vi "Find HTML Help Workshop Installation.vi"(8 "error in (no error)":errorcluster, 11 "Help Path":path) -> (0 "error out":errorcluster, 3 "Installation Path":string)   [LabVIEW 2015, in "HTML Help File Tools.lvlib"]
uses:
  HTML Help File Tools.lvlib
  <vilib>/registry/registry.llb/Registry RtKey.ctl
  <vilib>/registry/registry.llb/Registry SAM.ctl
  <vilib>/registry/registry.llb/Read Registry Value Simple STR.vi
  Log FGV Operation Modes.ctl
  Error Location.ctl
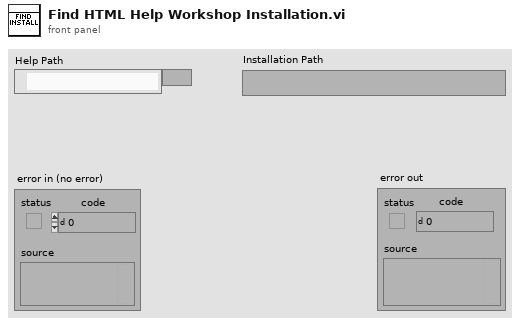
[diagram p1: front panel]
types:
  T1 = typedef "HTML Help File Tools.lvlib/Error Location.ctl" = enum16{"Delete tmp", "Compile HHP", "Find Install", "Create tmp", "Create HHP", "Find Help"}
  T2 = typedef "HTML Help File Tools.lvlib/Log FGV Operation Modes.ctl" = enum16{"Close", "Write", "Open File"}
  T3 = typedef "Registry SAM.ctl" = enum32{"KEY_QUERY_VALUE", "KEY_SET_VALUE", "KEY_CREATE_SUB_KEY", "KEY_ENUMERATE_SUB_KEYS", "KEY_NOTIFY", "KEY_CREATE_LINK", "KEY_READ", "KEY_WRITE", "KEY_ALL_ACCESS", "KEY_READ | KEY_WRITE"}
  T4 = typedef "Registry RtKey.ctl" = enum32{"HKEY_CLASSES_ROOT", "HKEY_CURRENT_USER", "HKEY_LOCAL_MACHINE", "HKEY_USERS", "HKEY_PERFORMANCE_DATA", "HKEY_CURRENT_CONFIG", "HKEY_DYN_DATA"}
  T5 = typedef "Registry refnum.ctl" = refnum<k1>
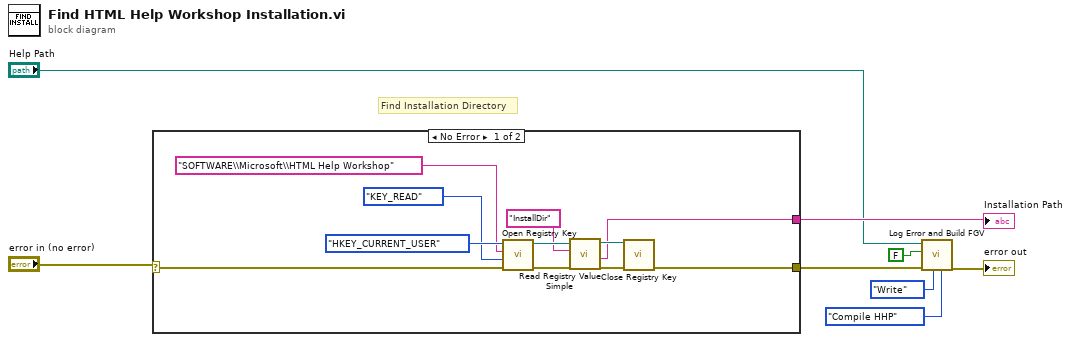
[diagram p0: block diagram]
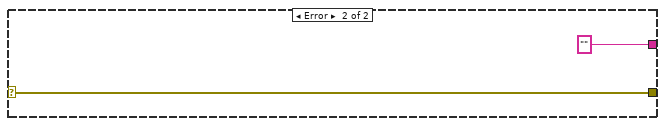
[diagram p2: hidden frame]
diagram:
  # "Find Installation Directory"
  n1 = case shown="No Error" "error in (no error)" {
    selector: "error in (no error)" -> [w11 w20]
    tunnel: [w10 w20] -> w6
    tunnel: [w9 "" ("String/Binary data")] -> w8
    frame No Error {
      n2 = call <vilib>:"Open Registry Key.vi"("error in (no error)"=w11, "security access mask (KEY_READ | KEY_WRITE)"=Registry_SAM."KEY_READ", "subkey"="SOFTWARE\\Microsoft\\HTML Help Workshop", "root key (HKEY_LOCAL_MACHINE)"=Registry_RtKey."HKEY_CURRENT_USER") -> ("error out"=w16:errorcluster, "refnum out"=w17:T5)  [unwired: 6 in]
      n3 = call-poly <vilib>:"Read Registry Value Simple.vi"("error in (no error)"=w16, "value"="InstallDir", "refnum"=w17) -> ("error out"=w13:errorcluster, "String/Binary data"=w9:string, "refnum out"=w12:T5)  [unwired: 3 in, 1 out]
      n4 = call <vilib>:"Close Registry Key.vi"("error in (no error)"=w13, "refnum"=w12) -> ("error out"=w10:errorcluster)  [unwired: 5 in]
    }
    frame Error {
    }
  }
  "Installation Path" <- w8
  n5 = call "Log Error and Build FGV.vi"("Error Location"=Error_Location."Compile HHP", "Operation Mode"=Log_FGV_Operation_Modes."Write", "error in"=w6, "Log Build Output?"=FALSE, "Help Documentation Path"="Help Path") -> ("error out"=→"error out":errorcluster)  [unwired: 6 in]
